vi "RT Create Target Disk Image Core.vi"(4 "file blacklist":string[](array[string]), 6 "image name":string, 8 "error in (no error)":errorcluster, 9 "allow overwrite? (F)":bool, 10 "base path":path, 11 "target address":string) -> (0 "error out":errorcluster, 2 "image path":path, 3 "target address out":string)   [LabVIEW 2017, in "NI_Real-Time Libraries.lvlib"]
doc: "LabVIEW no longer supports this VI. For information about replacing the RT Utility VIs, refer to ni.com/info and enter the Info Code RT_Utility_Replace. Copies the contents of the primary hard drive on the RT target to the local zip file you specify using the <B>image file path</B> input.\n\n<B>target address</B> specifies the IP address or DNS name of the target. \n\n<B>image file path</B> specifies the name and location of the RT target disk image on the local computer. To ensure compatibility, National Instruments recommends that you use a file name with a .zip extension. \n\n<B>allow overwrite?</B> specifies whether this VI can overwrite an existing file at the specified <B>image file path</B>. If <B>allow overwrite?</B> is TRUE, this VI overwrites the contents of <B>image file path</B>. If <B>allow overwrite?</B> is FALSE and <B>image file path</B> already exists on the local computer, this VI returns an error. \n\n<B>error in</B> describes error conditions that occur before this node runs. This input provides standard error in functionality. \n\n<B>file blacklist</B> specifies an array of file paths to exclude from the target image. To enable filtering through strict matching, the data type of this control is an array of strings rather than an array of paths. \n\n<B>target address out</B> returns the same address as <B>target address</B>. \n\n<B>image file path out</B> returns the same path as <B>image path</B>. \n\n<B>error out</B> contains error information. This output provides standard error out functionality. \n\n\nRT Create Target Disk Image Details\nThis VI stores the RT target disk image as a ZIP file. Use the RT Apply Target Disk Image VI to apply the disk images you create using this VI. This VI does not support disk images based on RT targets with multiple operating systems or multiple hard disk partitions."
uses:
  <vilib>/real-time/NI_Real-Time Libraries.lvlib
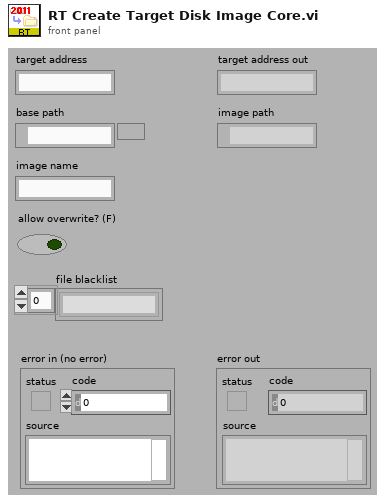
[diagram p1: front panel]
types:
  T1 = typedef "NI_FTP.lvlib/FTP Session.ctl" = refnum<k5>
  T2 = typedef "NI_Real-Time Libraries.lvlib/RT Target Information.ctl" = cluster{"IP settings":T3, "MAC address":string, "serial number":u32, "system state":string, "model name":string, "model code":string, "password protected restarts?":bool, "halt if TCP/IP fails?":bool, "locked?":bool, "use DHCP?":bool}
  T3 = typedef "NI_Real-Time Libraries.lvlib/IP Settings.ctl" = cluster{"IP address":string, "DNS name":string, "subnet mask":string, "gateway":string, "DNS server":string}
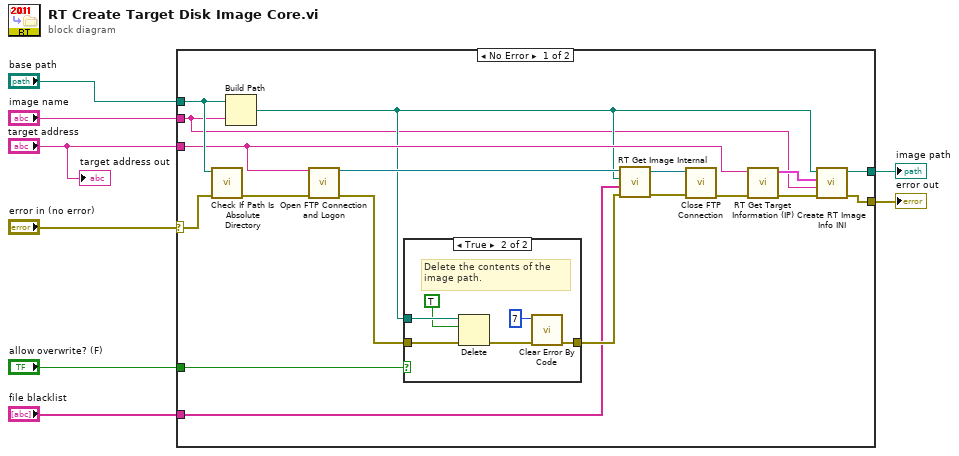
[diagram p0: block diagram]
diagram:
  n1 = case shown="No Error" "error in (no error)" {
    selector: "error in (no error)" -> [w21 w35]
    tunnel: [w25 w35] -> w6
    tunnel: "target address" -> [w19 _]
    tunnel: "base path" -> [w20 w34]
    tunnel: [w26 w34] -> w5
    tunnel: "image name" -> [w9 _]
    tunnel: "allow overwrite? (F)" -> [w24 _]
    tunnel: "file blacklist" -> [w11 _]
    frame No Error {
      n2 = call <vilib>:"Check If Path Is Absolute Directory.vi"("error in (no error)"=w21, "path"=w20) -> ("error out"=w18:errorcluster)  [unwired: 9 out]
      n3 = Build Path(base path=w20, name or relative path=w9) -> (appended path=w10:path)
      n4 = call <vilib>:"Open FTP Connection and Logon.vi"("address"=w19, "error in (no error)"=w18) -> ("ftp session out"=w12:T1, "error out"=w16:errorcluster)  [unwired: 3 in, 9 out]
      n5 = case shown="True" w24 {
        tunnel: [w27 w30] -> w15
        tunnel: w16 -> [w27 w32]
        tunnel: w10 -> [_ w33]
        frame False {
        }
        frame True {
          # "Delete the contents of the image path."
          n6 = Delete(path (use dialog)=w33, entire hierarchy (F)=TRUE, error in=w32) -> (error out=w29:errorcluster)  [unwired: 4 out]
          n7 = call <vilib>:"Clear Error By Code.vi"("error in (no error)"=w29, "Error Code"=7) -> ("error out"=w30:errorcluster)  [unwired: 9 out]
        }
      }
      n8 = call <vilib>:"RT Get Image Internal.vi"("error in (no error)"=w15, "blacklist file paths"=w11, "image path"=w10, "ftp session"=w12) -> ("error out"=w14:errorcluster, "ftp session out"=w13:T1)  [unwired: 6 out]
      n9 = call <vilib>:"Close FTP Connection.vi"("error in (no error)"=w14, "ftp session"=w13) -> ("error out"=w17:errorcluster)  [unwired: 9 out]
      n10 = call <vilib>:"RT Get Target Information (IP).vi"("error in (no error)"=w17, "target address"=w19) -> ("error out"=w22:errorcluster, "target information"=w23:T2)  [unwired: 1 in, 7 out]
      n11 = call <vilib>:"Create RT Image Info INI.vi"("error in (no error)"=w22, "image name"=w9, "RT target information"=w23, "image path"=w10) -> ("error out"=w25:errorcluster, "image path out"=w26:path)  [unwired: 6 out]
    }
    frame Error {
    }
  }
  "error out" <- w6
  "image path" <- w5
  "target address out" <- "target address"
